vi "MAD_Filename.vi"(8 "error in":errorcluster, 11 "XLS in":refnum<class "XLS.lvclass">) -> (0 "error out":errorcluster, 3 "XLS out":refnum<class "XLS.lvclass">)   [LabVIEW 2017, in "Report_lib.lvlib" / "XLS.lvclass"]
uses:
  XLS.lvclass
  I:/TEMP/Source/Classes/Log/Log.lvclass
  XLS.lvclass/XLS.ctl
  Log/Log.lvclass
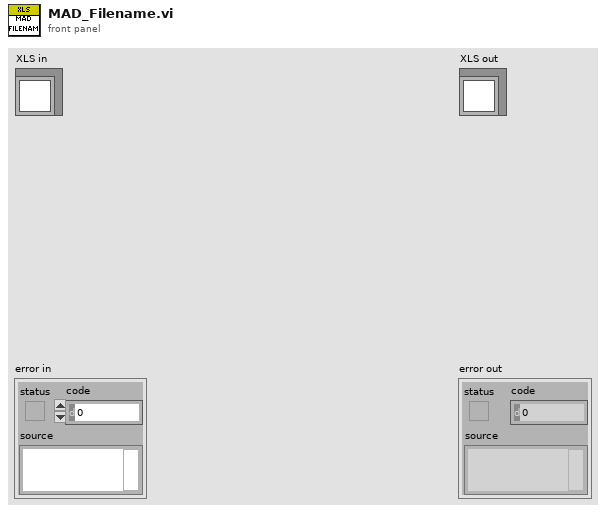
[diagram p1: front panel]
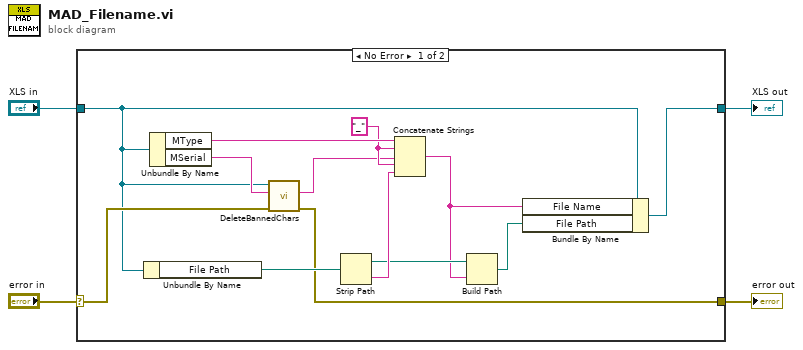
[diagram p0: block diagram]
diagram:
  n1 = case shown="No Error" "error in" {
    selector: "error in" -> [w6 w19]
    tunnel: [w9 w19] -> w3
    tunnel: [w10 w18] -> w1
    tunnel: "XLS in" -> [w5 w18]
    frame No Error {
      w15 = "_"
      n2 = Unbundle By Name(w5) -> ("File Path"=w17:path)
      n3 = Unbundle By Name(w5) -> ("MType"=w16:string, "MSerial"=w8:string)
      n4 = call "DeleteBannedChars.vi"("error in"=w6, "string in"=w8, "Log in"=w5) -> ("error out"=w9:errorcluster, "string out"=w7:string)  [unwired: 6 in, 1 out]
      n5 = Strip Path(path=w17) -> (stripped path=w13:path, name=w14:string)
      n6 = Concatenate Strings(w16, w15, w7, w15, w14) -> (w11:string)
      n7 = Build Path(base path=w13, name or relative path=w11) -> (appended path=w12:path)
      n8 = Bundle By Name(cluster=w5, "File Name"=w11, "File Path"=w12) -> (w10:refnum<class "XLS.lvclass">)
    }
    frame Error {
    }
  }
  "error out" <- w3
  "XLS out" <- w1
